vi "GetAccumulationConfig.vi"(7 "Qbus":refnum<class "Qbus.lvclass">, 8 "error in (no error)":errorcluster, 10 "data":T4, 11 "config":variant) -> (0 "error out":errorcluster, 1 "accumulation settings":T1, 2 "clear buffer":bool, 3 "config":variant, 4 "accumulation settings key":string, 5 "ok to start":bool)   [LabVIEW 2017, in "DataAccumulator.lvlib"]
uses:
  <vilib>/addons/InsightCM/Devices/Shared/Common/DataAccumulator/DataAccumulator.lvlib
  <vilib>/addons/InsightCM/Devices/Shared/Common/DataFlow/controls/Data.ctl
  <vilib>/addons/InsightCM/Utilities/DataAccessors/controls/wfmSGL_DVR.ctl
  <vilib>/addons/PointValueMap/controls/PointMap.ctl
  <vilib>/addons/InsightCM/Devices/Shared/Common/DataFlow/controls/Type.ctl
  <vilib>/addons/InsightCM/Devices/Shared/Common/DataAccumulator/controls/AccumulationSettings.ctl
  <vilib>/addons/InsightCM/Devices/Shared/Common/DataAccumulator/controls/accumulationType.ctl
  <vilib>/addons/InsightCM/Devices/Shared/Common/DVRBuffer/controls/BufferLocation.ctl
  <vilib>/addons/Qbus/Qbus.lvclass
  <vilib>/addons/InsightCM/Devices/Shared/Common/DataAccumulator/controls/config.ctl
  <vilib>/addons/InsightCM/Devices/Shared/Common/DeviceHealth/controls/deviceHealthTag.ctl
  <vilib>/addons/InsightCM/Devices/Shared/Common/DeviceHealth/controls/SystemHealthTagEnum.ctl
  <vilib>/addons/InsightCM/MessageBus/Base/controls/Tag.ctl
  <vilib>/addons/InsightCM/MessageBus/Base/controls/KeyValuePair.ctl
  <vilib>/addons/PointValueMap/subVIs/Point_Read_string.vi
  <vilib>/addons/PointValueMap/PointValueMap.lvlib
  <vilib>/addons/InsightCM/Devices/Shared/Common/DVRBuffer/DVRBuffer.lvlib
  <vilib>/addons/InsightCM/Devices/Shared/Common/DeviceHealth/DeviceHealth.lvlib
  <vilib>/addons/InsightCM/Devices/Shared/Common/DataFlow/DataFlow.lvlib
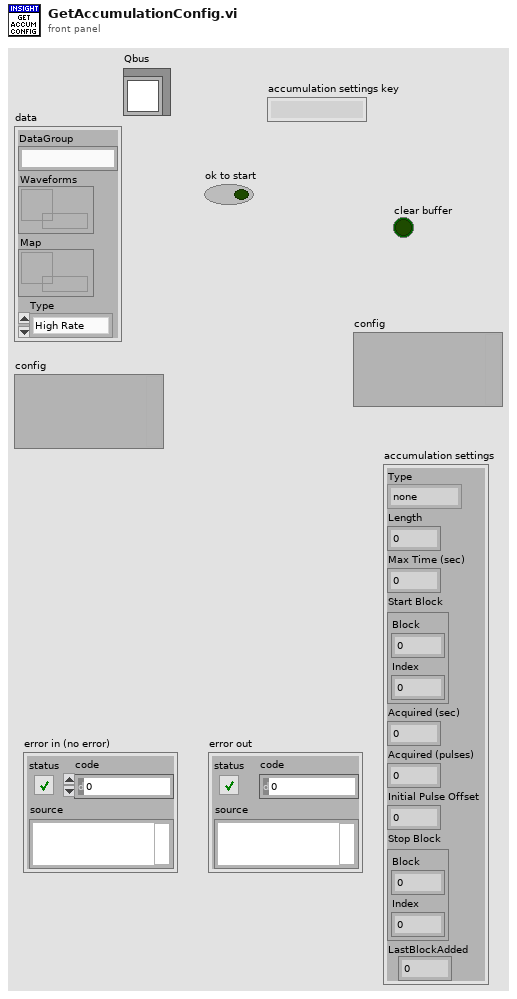
[diagram p1: front panel]
types:
  T1 = typedef "DataAccumulator.lvlib/AccumulationSettings.ctl" = cluster{"Type":T2, "Length":dbl, "Max Time (sec)":dbl, "Start Block":T3, "Acquired (sec)":dbl, "Acquired (pulses)":i32, "Initial Pulse Offset":dbl, "Stop Block":T3, "LastBlockAdded":u32}
  T2 = typedef "DataAccumulator.lvlib/accumulationType.ctl" = enum16{"none", "seconds", "revolutions"}
  T3 = typedef "DVRBuffer.lvlib/BufferLocation.ctl" = cluster{"Block":u32, "Index":i32}
  T4 = typedef "DataFlow.lvlib/Data.ctl" = cluster{"DataGroup":string, "Waveforms":T5, "Map":T6, "Type":T7}
  T5 = typedef "wfmSGL_DVR.ctl" = refnum<data-value>
  T6 = typedef "PointValueMap.lvlib/PointMap.ctl" = refnum<data-value>
  T7 = typedef "DataFlow.lvlib/Type.ctl" = enum16{"High Rate", "Low Rate", "Burst Mode"}
  T8 = typedef "DataAccumulator.lvlib/config.ctl" = cluster{"Group":string, "BlockComplete":bool, "Ok To Start":bool, "Speed Ref Chan":string, "Current OpState":string, "MaxLowRateCPU(%)":dbl, "MaxLowRateMem(%)":dbl, "LowRateCount":i32, "LowRateCountTag":T9}
  T9 = typedef "DeviceHealth.lvlib/deviceHealthTag.ctl" = cluster{"SystemTags":T10, "TagId":string, "Tag":T11}
  T10 = typedef "DeviceHealth.lvlib/SystemHealthTagEnum.ctl" = enum16{"CPU Utilization", "Memory Utilization", "Disk Utilization", "Total Physical Memory", "Primary Disk Free", "Chassis Temperature", "LowRateCount"}
  T11 = typedef "Tag.ctl" = cluster{"Id":string, "Path":string, "Name":string, "Datatype":string, "Props":T12[], "Keywords":string[]}
  T12 = typedef "KeyValuePair.ctl" = cluster{"Key":string, "Value":string}
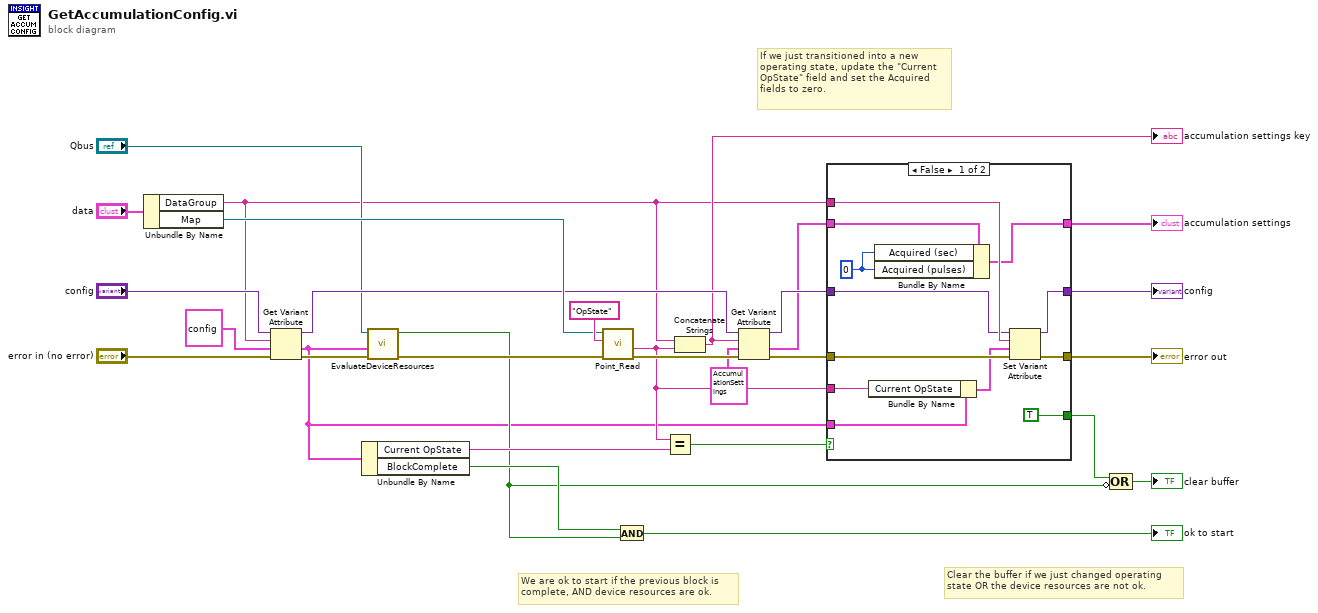
[diagram p0: block diagram]
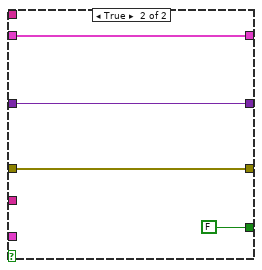
[diagram p2: hidden frame]
diagram:
  # "Clear the buffer if we just changed operating\nstate OR the device resources are not ok."
  # "We are ok to start if the previous block is \ncomplete, AND device resources are ok."
  # "If we just transitioned into a new\noperating state, update the \"Current\nOpState\" field and set the Acquired\nfields to zero."
  n1 = Unbundle By Name("data") -> ("DataGroup"=w2:string, "Map"=w27:T6)
  n2 = Get Variant Attribute(Variant="config", name=w2, default value (empty Variant)=T8 {"Group"="", "BlockComplete"=FALSE, "Ok To Start"=FALSE, "Speed Ref Chan"="", "Current OpState"="", "MaxLowRateCPU(%)"=0.0, "MaxLowRateMem(%)"=0.0, "LowRateCount"=0, "LowRateCountTag"={"SystemTags"=enum."CPU Utilization", "TagId"="", "Tag"={"Id"="", "Path"="", "Name"="", "Datatype"="", "Props"=[], "Keywords"=[]}}} ("Config"), error in="error in (no error)") -> (duplicate Variant=w26:variant, value=w1:T8, error out=w11:errorcluster)  [unwired: 1 out]
  n3 = Unbundle By Name(w1) -> ("Current OpState"=w22:string, "BlockComplete"=w13:bool)
  n4 = call <vilib>:"EvaluateDeviceResources.vi"("error in (no error)"=w11, "accumulation config"=w1, "Qbus"="Qbus") -> ("error out"=w12:errorcluster, "device resources ok"=w8:bool)  [unwired: 7 in]
  n5 = call-poly <vilib>:"Point_Read.vi"("Error In"=w12, "Tag"="OpState", "Map"=w27) -> ("Error Out"=w25:errorcluster, "Value"=w19:string)  [unwired: 3 in, 4 out]
  n6 = And(x=w13, y=w8) -> (x .and. y?=→"ok to start":bool)
  n7 = Equal?(x=w19, y=w22) -> (x = y?=w18:bool)
  n8 = Concatenate Strings(w2, w19) -> (w24:string)
  "accumulation settings key" <- w24
  n9 = Get Variant Attribute(Variant=w26, name=w24, default value (empty Variant)=T1 {"Type"=enum."none", "Length"=0.0, "Max Time (sec)"=0.0, "Start Block"={"Block"=0, "Index"=0}, "Acquired (sec)"=0.0, "Acquired (pulses)"=0, "Initial Pulse Offset"=0.0, "Stop Block"={"Block"=0, "Index"=0}, "LastBlockAdded"=0} ("Accumulation Settings"), error in=w25) -> (duplicate Variant=w17:variant, value=w15:T1, error out=w21:errorcluster)  [unwired: 1 out]
  n10 = case shown="False" w18 {
    tunnel: w21 -> [w41 w45]
    tunnel: [w40 w45] -> w20
    tunnel: w1 -> [w39 _]
    tunnel: w19 -> [w38 _]
    tunnel: w2 -> [w36 _]
    tunnel: [TRUE FALSE] -> w9
    tunnel: w17 -> [w34 w43]
    tunnel: [w33 w43] -> w16
    tunnel: w15 -> [w32 w42]
    tunnel: [w31 w42] -> w14
    frame False {
      w30 = 0 ("Acquired (pulses)")
      n11 = Bundle By Name(cluster=w39, "Current OpState"=w38) -> (w37:T8)
      n12 = Bundle By Name(cluster=w32, "Acquired (sec)"=w30, "Acquired (pulses)"=w30) -> (w31:T1)
      n13 = Set Variant Attribute(Variant=w34, name=w36, value=w37, error in=w41) -> (Variant out=w33:variant, error out=w40:errorcluster)  [unwired: 1 out]
    }
    frame True {
    }
  }
  "accumulation settings" <- w14
  "config" <- w16
  "error out" <- w20
  n14 = Compound Arithmetic op=OR(w9, invert w8) -> (→"clear buffer":bool)
